vi "Auto Drive XY.vi"(0 "RobotDriveDevRef In":T2={"DevStatus"={"status"=FALSE, "code"=0, "source"=""}, "Motors[]"=[], "Square Inputs"=FALSE, "Max Output"=1.0}, 1 "Angle Offset":dbl, 2 "Auto":string, 3 "Movement":dbl=-1.0, 5 "Motor Output Range X":cluster{"output high":dbl, "output low":dbl}={"output high"=0.7, "output low"=-0.7}, 7 "PID Gains X":T1={"proportional gain (Kc)"=0.07, "integral time (Ti, min)"=0.0, "derivative time (Td, min)"=0.0}, 9 "Distance (in)":dbl=15.0 format="%#_13g", 11 "Time to Settle (ms)":u32=50, 12 "Min Time (ms)":u32=250, 13 "PID Gains Y":T1={"proportional gain (Kc)"=0.07, "integral time (Ti, min)"=0.0, "derivative time (Td, min)"=0.0}, 14 "Motor Output Range Y":cluster{"output high":dbl, "output low":dbl}={"output high"=0.7, "output low"=-0.7}, 15 "Max Time (ms)":u32=15000) -> (4 "RobotDriveDevRef Out":T2={"DevStatus"={"status"=FALSE, "code"=0, "source"=""}, "Motors[]"=[], "Square Inputs"=FALSE, "Max Output"=1.0})   [LabVIEW 2017]
uses:
  <vilib>/Rock Robotics/WPI/RobotDrive/WPI_RobotDriveDevRef.ctl
  <vilib>/Rock Robotics/WPI/MotorControl/WPI_MotorControlDeviceRef.ctl
  <vilib>/Rock Robotics/WPI/MotorControl/WPI_MotorControlType.ctl
  <vilib>/Rock Robotics/SystemInterfaces/DIO/FPGA_DIOPWMChannel.ctl
  <vilib>/Rock Robotics/WPI/PWM/WPI_PWMDeadband.ctl
  <vilib>/Rock Robotics/SystemInterfaces/DIO/FPGA_DIOChannel.ctl
  <vilib>/Rock Robotics/WPI/Solenoid/WPI_SolenoidValue.ctl
  Globals/Robot Global Data.vi
  <vilib>/addons/control/pid/pid.llb/PID (DBL).vi
  <vilib>/Rock Robotics/WPI/RobotDrive/WPI_RobotDriveArcadeDrive_Standard(NoSaturation).vi
  <vilib>/addons/control/pid/NI_PID_pid.lvlib
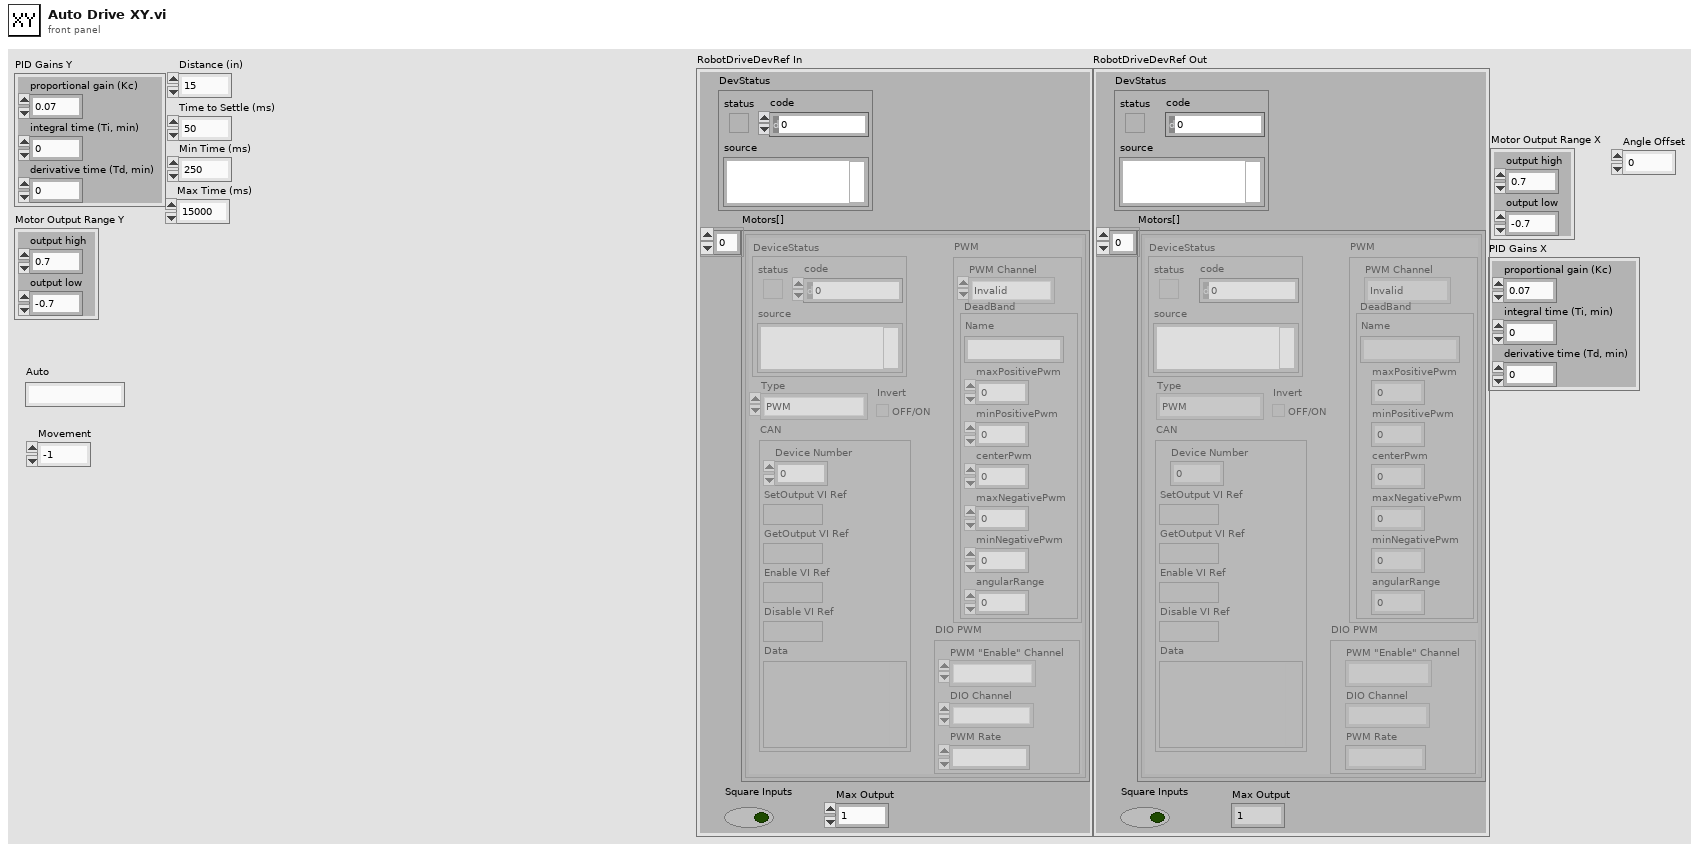
[diagram p1: front panel]
types:
  T1 = cluster{"proportional gain (Kc)":dbl, "integral time (Ti, min)":dbl, "derivative time (Td, min)":dbl}
  T2 = typedef "WPI_RobotDriveDevRef.ctl" = cluster{"DevStatus":errorcluster, "Motors[]":T3[], "Square Inputs":bool, "Max Output":dbl}
  T3 = typedef "WPI_MotorControlDeviceRef.ctl" = cluster{"DeviceStatus":errorcluster, "Type":T4, "PWM":cluster{"PWM Channel":T5, "DeadBand":T6}, "CAN":cluster{"Device Number":u8, "SetOutput VI Ref":variant, "GetOutput VI Ref":variant, "Enable VI Ref":variant, "Disable VI Ref":variant, "Data":variant}, "Invert":bool, "DIO PWM":cluster{"PWM \"Enable\" Channel":T5, "DIOChannel":T7, "PWM Rate":dbl}}
  T4 = typedef "WPI_MotorControlType.ctl" = enum16{"PWM", "CAN", "DIO PWM"}
  T5 = typedef "FPGA_DIOPWMChannel.ctl" = enum8{"PWM 0", "PWM 1", "PWM 2", "PWM 3", "PWM 4", "PWM 5", "PWM 6", "PWM 7", "PWM 8", "PWM 9", "PWM MXP 0", "PWM MXP 1", "PWM MXP 2", "PWM MXP 3", "PWM MXP 4", "PWM MXP 5", "PWM MXP 6", "PWM MXP 7", "PWM MXP 8", "PWM MXP 9", "Invalid"}
  T6 = typedef "WPI_PWMDeadband.ctl" = cluster{"Name":string, "maxPositivePwm":i32, "minPositivePwm":i32, "centerPwm":i32, "maxNegativePwm":i32, "minNegativePwm":i32, "angularRange":u16}
  T7 = typedef "FPGA_DIOChannel.ctl" = enum8{"DIO 0", "DIO 1", "DIO 2", "DIO 3", "DIO 4", "DIO 5", "DIO 6", "DIO 7", "DIO 8", "DIO 9", "DIO MXP 0", "DIO MXP 1", "DIO MXP 2", "DIO MXP 3", "DIO MXP 4", "DIO MXP 5", "DIO MXP 6", "DIO MXP 7", "DIO MXP 8", "DIO MXP 9", "DIO MXP 10", "DIO MXP 11", "DIO MXP 12", "DIO MXP 13", "DIO MXP 14", "DIO MXP 15", "SPI Port CS1", "SPI Port CS2", "SPI Port CS3", "SPI Port MISO", "SPI Port MOSI", "Invalid"}
  T8 = typedef "WPI_SolenoidValue.ctl" = enum16{"Off", "On", "Forward", "Reverse"}
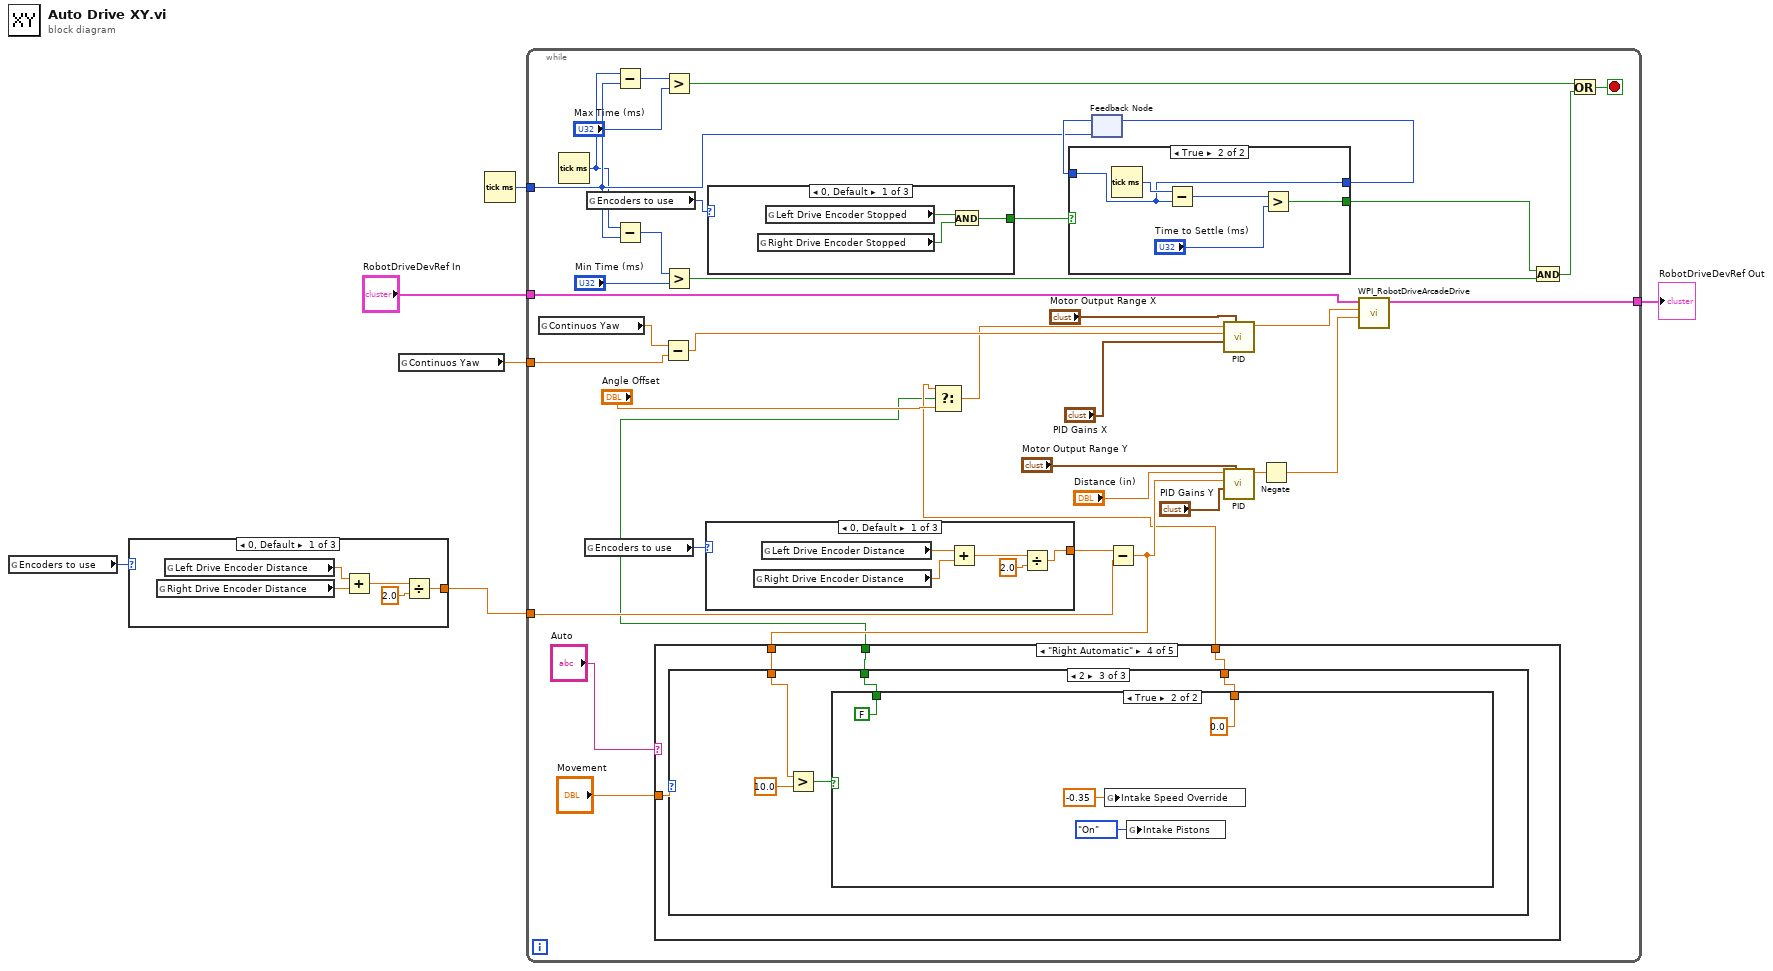
[diagram p0: block diagram]
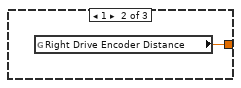
[diagram p2: hidden frame]
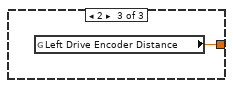
[diagram p3: hidden frame]
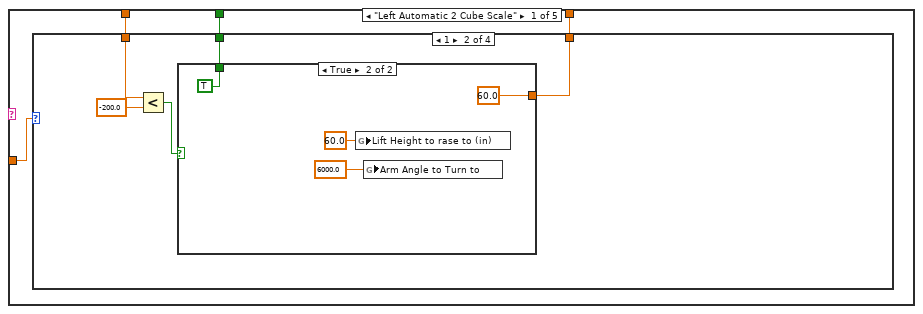
[diagram p4: hidden frame]
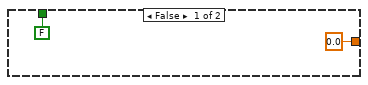
[diagram p6: hidden frame]
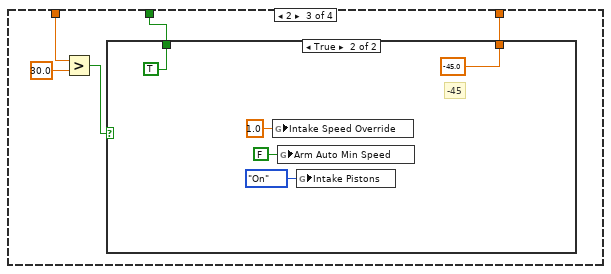
[diagram p7: hidden frame]
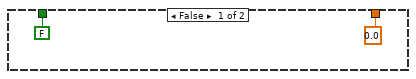
[diagram p8: hidden frame]
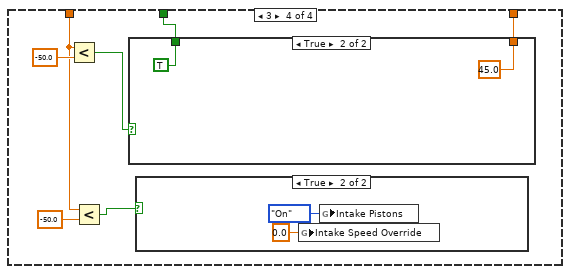
[diagram p9: hidden frame]
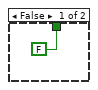
[diagram p11: hidden frame]
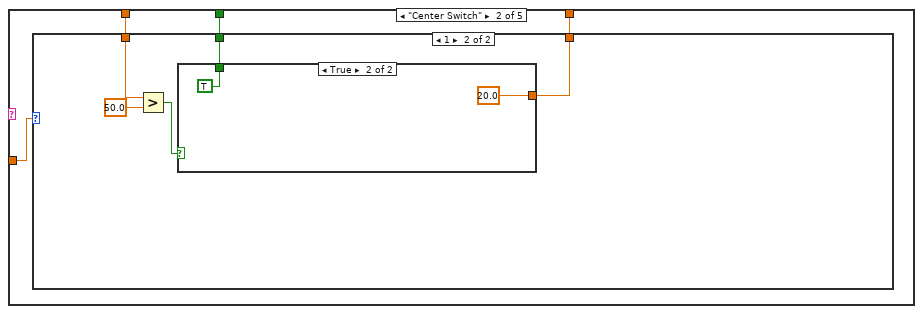
[diagram p12: hidden frame]
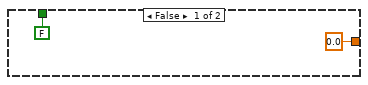
[diagram p14: hidden frame]
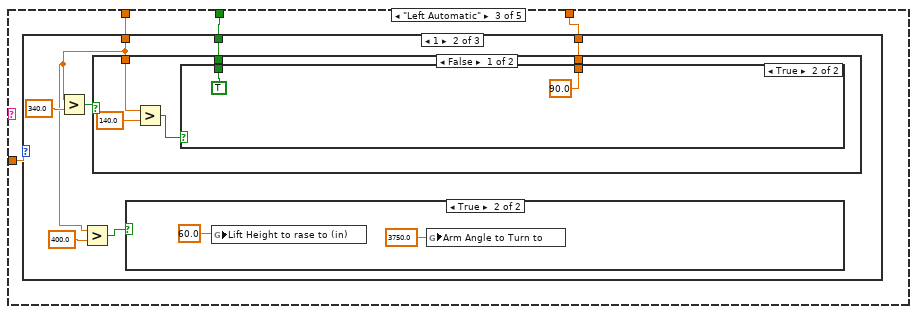
[diagram p15: hidden frame]
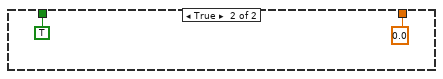
[diagram p19: hidden frame]
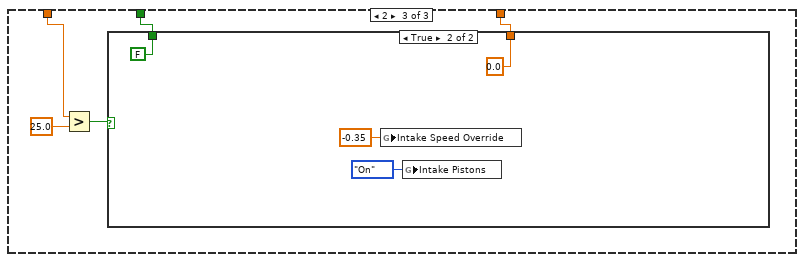
[diagram p20: hidden frame]
diagram:
  n1 = global read "Robot Global Data.vi" "Encoders to use"() -> (w2:u16)
  n2 = case shown="0, Default" w2 {
    tunnel: [w7 w12 w13] -> w6
    frame 0, Default {
      n3 = global read "Robot Global Data.vi" "Right Drive Encoder Distance"() -> (w10:dbl)
      n4 = global read "Robot Global Data.vi" "Left Drive Encoder Distance"() -> (w11:dbl)
      n5 = Add(x=w11, y=w10) -> (x+y=w9:dbl)
      n6 = Divide(x=w9, y=2.0) -> (x/y=w7:dbl)
    }
    frame 1 {
      n7 = global read "Robot Global Data.vi" "Right Drive Encoder Distance"() -> (w12:dbl)
    }
    frame 2 {
      n8 = global read "Robot Global Data.vi" "Left Drive Encoder Distance"() -> (w13:dbl)
    }
  }
  n9 = global read "Robot Global Data.vi" "Continuos Yaw"() -> (w1:dbl)
  n10 = Tick Count (ms)() -> (millisecond timer value=w5:u32)
  n11 = while {
    tunnel: "RobotDriveDevRef In" -> [w48]
    tunnel: w6 -> [w43]
    tunnel: w5 -> [w32]
    tunnel: [w42] -> w4
    tunnel: w1 -> [w22]
    stop <- w35 stop-if-true
    n12 = global read "Robot Global Data.vi" "Continuos Yaw"() -> (w23:dbl)
    n13 = Tick Count (ms)() -> (millisecond timer value=w31:u32)
    n14 = global read "Robot Global Data.vi" "Encoders to use"() -> (w30:u16)
    n15 = global read "Robot Global Data.vi" "Encoders to use"() -> (w28:u16)
    n16 = Subtract(x=w31, y=w32) -> (x-y=w36:u32)
    n17 = Subtract(x=w31, y=w32) -> (x-y=w41:u32)
    n18 = Subtract(x=w23, y=w22) -> (x-y=w21:dbl)
    n19 = Greater?(x=w36, y="Max Time (ms)") -> (0:w33:bool)
    n20 = Greater?(x=w41, y="Min Time (ms)") -> (0:w38:bool)
    n21 = case shown="0, Default" w30 {
      tunnel: [w173 w178 w179] -> w29
      frame 0, Default {
        n22 = global read "Robot Global Data.vi" "Right Drive Encoder Distance"() -> (w176:dbl)
        n23 = global read "Robot Global Data.vi" "Left Drive Encoder Distance"() -> (w177:dbl)
        n24 = Add(x=w177, y=w176) -> (x+y=w175:dbl)
        n25 = Divide(x=w175, y=2.0) -> (x/y=w173:dbl)
      }
      frame 1 {
        n26 = global read "Robot Global Data.vi" "Right Drive Encoder Distance"() -> (w178:dbl)
      }
      frame 2 {
        n27 = global read "Robot Global Data.vi" "Left Drive Encoder Distance"() -> (w179:dbl)
      }
    }
    n28 = case shown="0, Default" w28 {
      tunnel: [w170 w171 w172] -> w27
      frame 0, Default {
        n29 = global read "Robot Global Data.vi" "Right Drive Encoder Stopped"() -> (w168:bool)
        n30 = global read "Robot Global Data.vi" "Left Drive Encoder Stopped"() -> (w169:bool)
        n31 = And(x=w169, y=w168) -> (x .and. y?=w170:bool)
      }
      frame 1 {
        n32 = global read "Robot Global Data.vi" "Right Drive Encoder Stopped"() -> (w171:bool)
      }
      frame 2 {
        n33 = global read "Robot Global Data.vi" "Left Drive Encoder Stopped"() -> (w172:bool)
      }
    }
    n34 = feedback #1(w32) -> (w44:u32)
    n35 = case shown="True" w27 {
      tunnel: w44 -> [_ w185]
      tunnel: [w181 w185] -> w45
      tunnel: [FALSE w182] -> w39
      frame False {
        n36 = Tick Count (ms)() -> (millisecond timer value=w181:u32)
      }
      frame True {
        n37 = Tick Count (ms)() -> (millisecond timer value=w186:u32)
        n38 = Subtract(x=w186, y=w185) -> (x-y=w184:u32)
        n39 = Greater?(x=w184, y="Time to Settle (ms)") -> (0:w182:bool)
      }
    }
    n40 = feedback-in #1(w45) -> ()
    n41 = Subtract(x=w29, y=w43) -> (x-y=w18:dbl)
    n42 = case shown="\"Right Automatic\"" "Auto" {
      tunnel: "Movement" -> [w55 w94 w107 w138 _]
      tunnel: w18 -> [w54 w93 w106 w137 _]
      tunnel: [w53 w92 w104 w135 0.0 ("Intake Speed Override")] -> w15
      tunnel: [w52 w91 w105 w136 FALSE] -> w14
      frame "Left Automatic 2 Cube Scale" {
        n43 = case shown="1" w55 {
          tunnel: w54 -> [_ w60 w71 w80]
          tunnel: [_ w57 w68 w83] -> w53
          tunnel: [_ w56 w67 w82] -> w52
          frame -1, Default {
          }
          frame 1 {
            n44 = Less?(x=w60, y=-200.0) -> (x < y?=w58:bool)
            n45 = case shown="True" w58 {
              tunnel: [0.0 60.0] -> w57
              tunnel: [FALSE TRUE] -> w56
              frame False {
              }
              frame True {
                n46 = global write "Robot Global Data.vi" "Lift Height to rase to (in)"(60.0 ("Lift Height to rase to (in)")) -> ()
                n47 = global write "Robot Global Data.vi" "Arm Angle to Turn to"(6000.0 ("Lift Height to rase to (in)")) -> ()
              }
            }
          }
          frame 2 {
            n48 = Greater?(x=w71, y=30.0) -> (0:w69:bool)
            n49 = case shown="True" w69 {
              tunnel: [0.0 ("Intake Speed Override") -45.0 ("Intake Speed Override")] -> w68
              tunnel: [FALSE TRUE] -> w67
              frame False {
              }
              frame True {
                # "-45"
                n50 = global write "Robot Global Data.vi" "Intake Speed Override"(1.0 ("Intake Speed Override")) -> ()
                n51 = global write "Robot Global Data.vi" "Arm Auto Min Speed"(FALSE ("Arm Auto Min Speed")) -> ()
                n52 = global write "Robot Global Data.vi" "Intake Pistons"(WPI_SolenoidValue."On" ("Intake Pistons")) -> ()
              }
            }
          }
          frame 3 {
            n53 = Less?(x=w80, y=-50.0) -> (x < y?=w84:bool)
            n54 = Less?(x=w80, y=-50.0) -> (x < y?=w79:bool)
            n55 = case shown="True" w84 {
              tunnel: [_ 45.0] -> w83
              tunnel: [FALSE TRUE] -> w82
              frame False {
              }
              frame True {
              }
            }
            n56 = case shown="True" w79 {
              frame False {
              }
              frame True {
                n57 = global write "Robot Global Data.vi" "Intake Speed Override"(0.0 ("Intake Speed Override")) -> ()
                n58 = global write "Robot Global Data.vi" "Intake Pistons"(WPI_SolenoidValue."On" ("Intake Pistons")) -> ()
              }
            }
          }
        }
      }
      frame "Center Switch" {
        n59 = case shown="1" w94 {
          tunnel: w93 -> [_ w99]
          tunnel: [_ w96] -> w92
          tunnel: [_ w95] -> w91
          frame -1, Default {
          }
          frame 1 {
            n60 = Greater?(x=w99, y=50.0) -> (0:w97:bool)
            n61 = case shown="True" w97 {
              tunnel: [0.0 20.0] -> w96
              tunnel: [FALSE TRUE] -> w95
              frame False {
              }
              frame True {
              }
            }
          }
        }
      }
      frame "Left Automatic" {
        n62 = case shown="1" w107 {
          tunnel: w106 -> [_ w109 w130]
          tunnel: [_ w114 w127] -> w105
          tunnel: [_ w113 w126] -> w104
          frame -1, Default {
          }
          frame 1 {
            n63 = Greater?(x=w109, y=340.0) -> (0:w111:bool)
            n64 = Greater?(x=w109, y=400.0) -> (0:w108:bool)
            n65 = case shown="False" w111 {
              tunnel: w109 -> [w121 _]
              tunnel: [w118 TRUE] -> w114
              tunnel: [w117 0.0] -> w113
              frame False {
                n66 = Greater?(x=w121, y=140.0) -> (0:w119:bool)
                n67 = case shown="True" w119 {
                  tunnel: [_ TRUE] -> w118
                  tunnel: [_ 90.0] -> w117
                  frame False {
                  }
                  frame True {
                  }
                }
              }
              frame True {
              }
            }
            n68 = case shown="True" w108 {
              frame False {
              }
              frame True {
                n69 = global write "Robot Global Data.vi" "Lift Height to rase to (in)"(60.0 ("Arm Angle to Turn to")) -> ()
                n70 = global write "Robot Global Data.vi" "Arm Angle to Turn to"(3750.0 ("Arm Angle to Turn to")) -> ()
              }
            }
          }
          frame 2 {
            n71 = Greater?(x=w130, y=25.0) -> (0:w129:bool)
            n72 = case shown="True" w129 {
              tunnel: [_ FALSE] -> w127
              tunnel: [_ 0.0] -> w126
              frame False {
              }
              frame True {
                n73 = global write "Robot Global Data.vi" "Intake Speed Override"(-0.35 ("Intake Speed Override")) -> ()
                n74 = global write "Robot Global Data.vi" "Intake Pistons"(WPI_SolenoidValue."On" ("Intake Pistons")) -> ()
              }
            }
          }
        }
      }
      frame "Right Automatic" {
        n75 = case shown="2" w138 {
          tunnel: w137 -> [_ w140 w161]
          tunnel: [_ w145 w158] -> w136
          tunnel: [_ w144 w157] -> w135
          frame -1, Default {
          }
          frame 1 {
            n76 = Greater?(x=w140, y=310.0) -> (0:w142:bool)
            n77 = Greater?(x=w140, y=350.0) -> (0:w139:bool)
            n78 = case shown="False" w142 {
              tunnel: w140 -> [w152 _]
              tunnel: [w149 TRUE] -> w145
              tunnel: [w148 0.0] -> w144
              frame False {
                n79 = Greater?(x=w152, y=140.0) -> (0:w150:bool)
                n80 = case shown="True" w150 {
                  tunnel: [_ TRUE] -> w149
                  tunnel: [_ -90.0] -> w148
                  frame False {
                  }
                  frame True {
                  }
                }
              }
              frame True {
              }
            }
            n81 = case shown="True" w139 {
              frame False {
              }
              frame True {
                n82 = global write "Robot Global Data.vi" "Lift Height to rase to (in)"(60.0 ("Arm Angle to Turn to")) -> ()
                n83 = global write "Robot Global Data.vi" "Arm Angle to Turn to"(3750.0 ("Arm Angle to Turn to")) -> ()
              }
            }
          }
          frame 2 {
            n84 = Greater?(x=w161, y=10.0) -> (0:w160:bool)
            n85 = case shown="True" w160 {
              tunnel: [_ FALSE] -> w158
              tunnel: [_ 0.0] -> w157
              frame False {
              }
              frame True {
                n86 = global write "Robot Global Data.vi" "Intake Speed Override"(-0.35 ("Intake Speed Override")) -> ()
                n87 = global write "Robot Global Data.vi" "Intake Pistons"(WPI_SolenoidValue."On" ("Intake Pistons")) -> ()
              }
            }
          }
        }
      }
      frame "", Default {
      }
    }
    n88 = Select(t=w15, s=w14, f="Angle Offset") -> (s? t:f=w17:dbl)
    n89 = call-poly <vilib>:"PID.vi"("output range"="Motor Output Range X", "PID gains"="PID Gains X", "process variable"=w21, "setpoint"=w17) -> ("output"=w26:dbl)  [unwired: 6 in, 1 out]
    n90 = call-poly <vilib>:"PID.vi"("output range"="Motor Output Range Y", "PID gains"="PID Gains Y", "process variable"=w18, "setpoint"="Distance (in)") -> ("output"=w46:dbl)  [unwired: 6 in, 1 out]
    n91 = Negate(x=w46) -> (-x=w47:dbl)
    n92 = call-poly <vilib>:"WPI_RobotDriveArcadeDrive.vi"("Y axis value"=w47, "X axis value"=w26, "RobotDriveDevRef"=w48) -> ("RobotDriveDevRef"=w42:T2)  [unwired: 6 in, 2 out]
    n93 = And(x=w39, y=w38) -> (x .and. y?=w34:bool)
    n94 = Or(x=w33, y=w34) -> (x .or. y?=w35:bool)
  }
  "RobotDriveDevRef Out" <- w4
